vi "create_data_file.vi"(8 "timestamp":string, 9 "LED current (A)":string, 10 "Device details":T1={"Device label"="", "Pixel"=enum."1", "Area (cm^2)"=0.0}, 11 "experiment folder":path) -> (3 "Filepath out":path)   [LabVIEW 2018]
uses:
  typedefs/device_details.ctl
  <vilib>/Utility/file.llb/Write Delimited Spreadsheet (string).vi
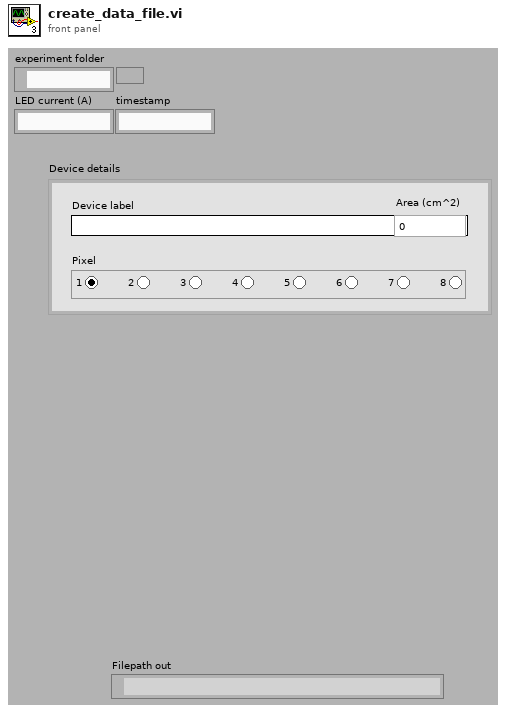
[diagram p1: front panel]
types:
  T1 = typedef "device_details.ctl" = cluster{"Device label":string, "Pixel":enum32{"No Selection", "1", "2", "3", "4", "5", "6", "7", "8"}, "Area (cm^2)":dbl}
  T2 = enum32{"No Selection", "1", "2", "3", "4", "5", "6", "7", "8"}
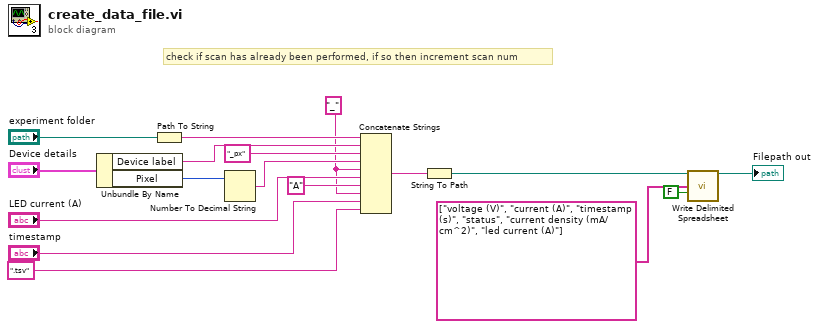
[diagram p0: block diagram]
diagram:
  w4 = "_"
  # "check if scan has already been performed, if so then increment scan num"
  n1 = Unbundle By Name("Device details") -> ("Device label"=w7:string, "Pixel"=w9:T2)
  n2 = Path To String(path="experiment folder") -> (string=w17:string)
  n3 = Number To Decimal String(number=w9) -> (decimal integer string=w8:string)  [unwired: 1 in]
  n4 = Concatenate Strings(w17, w7, "_px", w8, w4, "LED current (A)", "A" ("string"), w4, "timestamp", ".tsv" ("string")) -> (w13:string)
  n5 = String To Path(string=w13) -> (path=w2:path)
  n6 = call-poly <vilib>:"Write Delimited Spreadsheet.vi"("file path (dialog if empty)"=w2, "1D data"=string[] ["voltage (V)", "current (A)", "timestamp (s)", "status", "current density (mA/cm^2)", "led current (A)"] ("device headings"), "append to file? (new file:F)"=FALSE) -> ("new file path (Not A Path if cancelled)"=→"Filepath out":path)  [unwired: 11 in, 1 out]
